vi "Rotate from A to B.vi"(2 "Vector B":cluster{"X":sgl, "Y":sgl, "Z":sgl}, 3 "Vector A":cluster{"X":sgl, "Y":sgl, "Z":sgl}) -> (0 "Rotation.Angle":dbl, 1 "Rotation.Axis":cluster{"X":sgl, "Y":sgl, "Z":sgl})   [LabVIEW 2019]
doc: "This VI calculates the rotation axis and rotation angle from vector A to Vector B."
uses:
  <vilib>/Analysis/NI_AALPro.lvlib
  <vilib>/Analysis/_algsub.llb/Real Vector Norm.vi
  <vilib>/Analysis/NI_AALBase.lvlib
  <vilib>/Analysis/baseanly.llb/Real Dot Product.vi
panel:
  # "This VI calculates the rotation axis and rotation angle from vector A to Vector B."
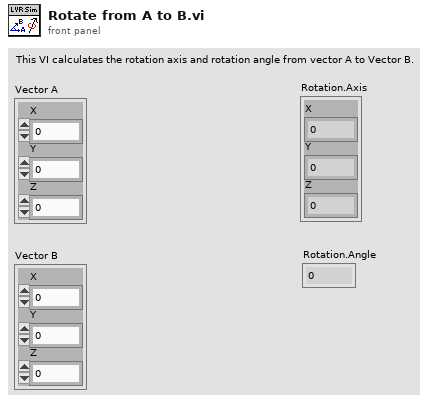
[diagram p1: front panel]
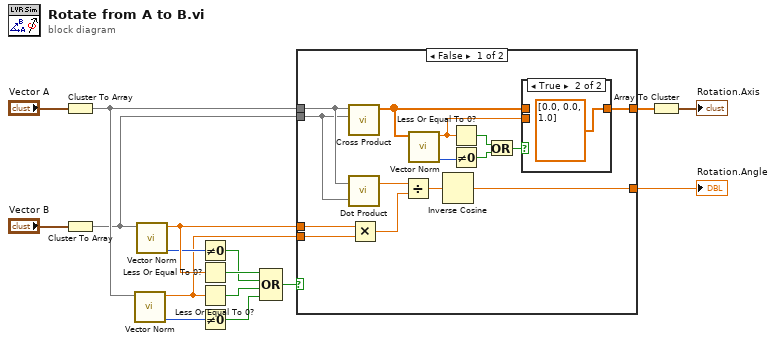
[diagram p0: block diagram]
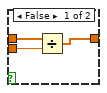
[diagram p2: hidden frame]
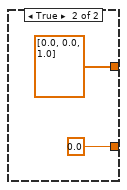
[diagram p3: hidden frame]
diagram:
  n1 = Cluster To Array(cluster="Vector A") -> (array=w14:sgl[])
  n2 = Cluster To Array(cluster="Vector B") -> (array=w13:sgl[])
  n3 = call-poly <vilib>:"Vector Norm.vi"("Input Vector"=w14) -> ("error"=w8:i32, "norm"=w9:dbl)  [unwired: 9 in]
  n4 = call-poly <vilib>:"Vector Norm.vi"("Input Vector"=w13) -> ("error"=w10:i32, "norm"=w11:dbl)  [unwired: 9 in]
  n5 = Not Equal To 0?(x=w10) -> (x != 0?=w6:bool)
  n6 = Less Or Equal To 0?(x=w11) -> (x <= 0?=w7:bool)
  n7 = Less Or Equal To 0?(x=w9) -> (x <= 0?=w5:bool)
  n8 = Not Equal To 0?(x=w8) -> (x != 0?=w4:bool)
  n9 = Compound Arithmetic op=OR(w7, w6, w5, w4) -> (w3:bool)
  n10 = case shown="False" w3 {
    tunnel: [w17 dbl[] [0.0, 0.0, 1.0]] -> w16
    tunnel: w14 -> [w30 _]
    tunnel: w13 -> [w29 _]
    tunnel: [w26 0.0] -> w12
    tunnel: w11 -> [w25 _]
    tunnel: w9 -> [w24 _]
    frame False {
      n11 = call <vilib>:"Cross Product.vi"("B Vector"=w29, "A Vector"=w30) -> ("Cross Product"=w19:dbl[])  [unwired: 8 in, 1 out]
      n12 = call-poly <vilib>:"Dot Product.vi"("Y Vector"=w29, "X Vector"=w30) -> ("X * Y"=w28:dbl)  [unwired: 1 out]
      n13 = Multiply(x=w25, y=w24) -> (x*y=w31:dbl)
      n14 = Divide(x=w28, y=w31) -> (x/y=w27:dbl)
      n15 = call-poly <vilib>:"Vector Norm.vi"("Input Vector"=w19) -> ("error"=w23:i32, "norm"=w18:dbl)  [unwired: 9 in]
      n16 = Inverse Cosine(1:w27) -> (0:w26:dbl)
      n17 = Less Or Equal To 0?(x=w18) -> (x <= 0?=w22:bool)
      n18 = Not Equal To 0?(x=w23) -> (x != 0?=w21:bool)
      n19 = Or(x=w22, y=w21) -> (x .or. y?=w20:bool)
      n20 = case shown="True" w20 {
        tunnel: w19 -> [w33 _]
        tunnel: w18 -> [w34 _]
        tunnel: [w32 dbl[] [0.0, 0.0, 1.0]] -> w17
        frame False {
          n21 = Divide(x=w33, y=w34) -> (x/y=w32:dbl[])
        }
        frame True {
        }
      }
    }
    frame True {
    }
  }
  "Rotation.Angle" <- w12
  n22 = Array To Cluster(array=w16) -> (cluster=→"Rotation.Axis":cluster{"[0]":dbl, "[1]":dbl, "[2]":dbl})
